vi "LWXPS_PositionerCompensationPositionFilterGet.vi"(8 "LabVIEW error IN":errorcluster, 9 "Filter Number":i32, 10 "Positioner Name":string, 11 "XPS Reference IN":refnum<k24>) -> (0 "XPS Error String":string, 1 "Damping Factor":dbl, 2 "Frequency":dbl, 3 "Returned error code":i32, 4 "LabVIEW error OUT":errorcluster, 5 "XPS Reference OUT":refnum<k24>)   [LabVIEW 2014]
uses:
  D:/XPSQ8_LabView_Library/Development/Source/Dll/Newport.XPS.CommandInterface.dll
  Dll/Newport.XPS.CommandInterface.dll
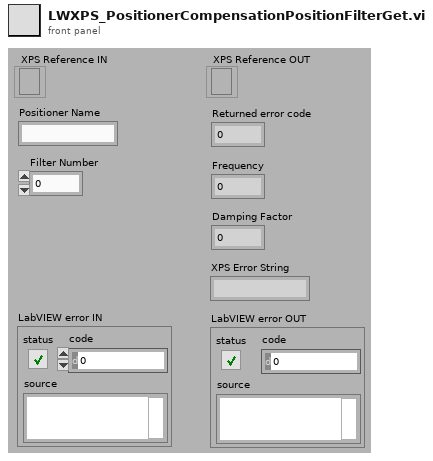
[diagram p1: front panel]
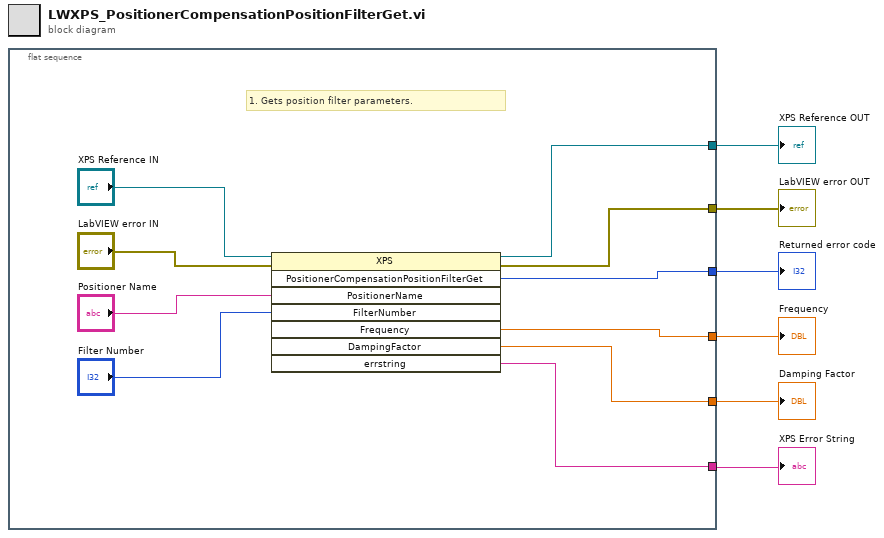
[diagram p0: block diagram]
diagram:
  n1 = flat-sequence {
    tunnel: [w14] -> w6
    tunnel: [w8] -> w5
    tunnel: [w15] -> w4
    tunnel: [w11] -> w3
    tunnel: [w10] -> w2
    tunnel: [w9] -> w1
    frame #0 {
      # "1. Gets position filter parameters."
      n2 = invoke class="XPS" method="PositionerCompensationPositionFilterGet"(reference="XPS Reference IN", error in="LabVIEW error IN", "PositionerName"="Positioner Name", "FilterNumber"="Filter Number") -> (reference out=w14:refnum<k24>, error out=w8:errorcluster, "PositionerCompensationPositionFilterGet"=w15:i32, "Frequency"=w11:dbl, "DampingFactor"=w10:dbl, "errstring"=w9:string)  [unwired: 4 in, 2 out]
    }
  }
  "XPS Error String" <- w1
  "XPS Reference OUT" <- w6
  "LabVIEW error OUT" <- w5
  "Returned error code" <- w4
  "Frequency" <- w3
  "Damping Factor" <- w2
